vi "Window call-Raw data viewer.vi"(8 "error in (no error)":errorcluster) -> (0 "error out":errorcluster)   [LabVIEW 2020]
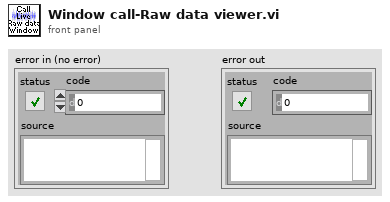
[diagram p1: front panel]
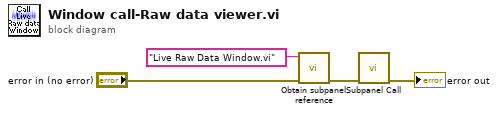
[diagram p0: block diagram]
diagram:
  n1 = call "Obtain subpanel reference.vi"("error in (no error)"="error in (no error)", "Subpanel VI name (plus \".vi\" file extension)"="Live Raw Data Window.vi" ("name or relative path")) -> ("error out"=w1:errorcluster)  [unwired: 8 in, 1 out]
  n2 = call "Subpanel Call.vi"("error in (no error)"=w1) -> ("error out"=→"error out":errorcluster)  [unwired: 10 in]
